vi "Scan Start Stimulus.vi"(8 "error in (no error)":errorcluster, 10 "Event ID (\"NONE\")":string="NONE", 11 "VISA resource name":refnum<visa-resource-name>) -> (0 "error out":errorcluster, 3 "VISA resource name out":refnum<visa-resource-name>)   [LabVIEW 2016, in "Keithley DMM6500 DAQ6500 Series.lvlib"]
doc: "Determines which event starts the scan."
uses:
  Keithley DMM6500 DAQ6500 Series.lvlib
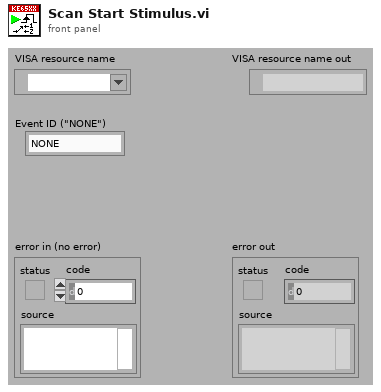
[diagram p1: front panel]
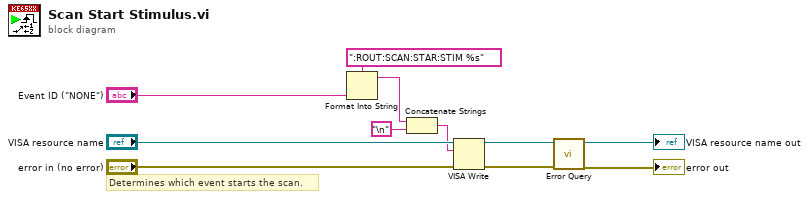
[diagram p0: block diagram]
diagram:
  # "Determines which event starts the scan."
  n1 = Format Into String(format string=":ROUT:SCAN:STAR:STIM %s", "Event ID (\"NONE\")") -> (resulting string=w2:string)  [unwired: 2 in, 1 out]
  n2 = Concatenate Strings(w2, "\n") -> (w3:string)
  n3 = VISA Write(VISA resource name="VISA resource name", write buffer=w3, error in (no error)="error in (no error)") -> (VISA resource name out=w8:refnum<visa-resource-name>, error out=w7:errorcluster)  [unwired: 1 out]
  n4 = call "Error Query.vi"("error in (no error)"=w7, "VISA resource name"=w8) -> ("error out"=→"error out":errorcluster, "VISA resource name out"=→"VISA resource name out":refnum<visa-resource-name>)  [unwired: 6 in, 2 out]
